vi "Bracket Deletion.vi"(0 "string input with brackets":string, 1 "error in (no error)":errorcluster) -> (2 "string output balanced":string, 3 "string output rest":string, 4 "error out":errorcluster)   [LabVIEW 2020, in "NI_Gmath.lvlib"]
uses:
  <vilib>/gmath/NI_Gmath.lvlib
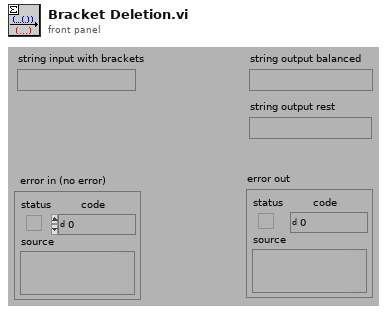
[diagram p1: front panel]
types:
  T1 = cluster{bool, i32, "string input with brackets":string}
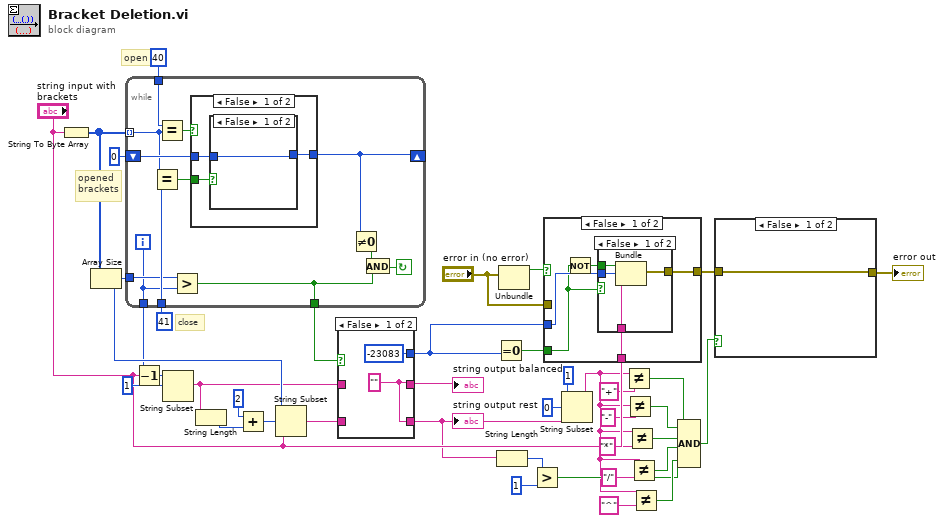
[diagram p0: block diagram]
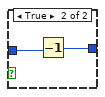
[diagram p2: hidden frame]
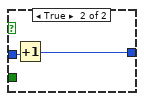
[diagram p3: hidden frame]
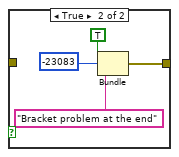
[diagram p4: hidden frame]
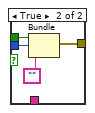
[diagram p5: hidden frame]
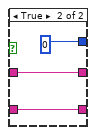
[diagram p7: hidden frame]
diagram:
  # "close"
  # "open"
  # "opened\nbrackets"
  n1 = String To Byte Array(string="string input with brackets") -> (unsigned byte array=w37:u8[])
  n2 = Array Size(array=w37) -> (size(s)=w36:i32)
  n3 = while {
    tunnel: [w41] -> w33
    tunnel: [w42] -> w25
    tunnel: w36 -> [w45]
    tunnel: 41 -> [w49]
    tunnel: 40 -> [w52]
    tunnel: w37 -> [w48] mode=indexing
    shift-left: 0 -> [w50]
    shift-right: [w46] -> _
    i -> [w41]
    stop <- w43 continue-if-true
    n4 = Equal?(x=w48, y=w49) -> (x = y?=w47:bool)
    n5 = Equal?(x=w52, y=w48) -> (x = y?=w51:bool)
    n6 = Greater?(x=w45, y=w41) -> (0:w42:bool)
    n7 = case shown="False" w51 {
      tunnel: w50 -> [w54 w60]
      tunnel: [w53 w59] -> w46
      tunnel: w47 -> [w55 _]
      frame False {
        n8 = case shown="False" w55 {
          tunnel: w54 -> [w56 w58]
          tunnel: [w56 w57] -> w53
          frame False {
          }
          frame True {
            n9 = Decrement(x=w58) -> (x-1=w57:i32)
          }
        }
      }
      frame True {
        n10 = Increment(x=w60) -> (x+1=w59:i32)
      }
    }
    n11 = Not Equal To 0?(x=w46) -> (x != 0?=w44:bool)
    n12 = And(x=w44, y=w42) -> (x .and. y?=w43:bool)
  }
  n13 = Decrement(x=w33) -> (x-1=w31:i32)
  n14 = String Subset(string="string input with brackets", offset (0)=1, length (rest)=w31) -> (substring=w35:string)
  n15 = String Length(string=w35) -> (length=w30:i32)
  n16 = Add(x=2, y=w30) -> (x+y=w28:i32)
  n17 = String Subset(string="string input with brackets", offset (0)=w28, length (rest)=w36) -> (substring=w34:string)
  n18 = case shown="False" w25 {
    tunnel: [-23083 0] -> w24
    tunnel: w35 -> [_ w64]
    tunnel: [w61 w64] -> w23
    tunnel: w34 -> [_ w63]
    tunnel: [w61 w63] -> w20
    frame False {
      w61 = ""
    }
    frame True {
    }
  }
  "string output balanced" <- w23
  "string output rest" <- w20
  n19 = Equal To 0?(x=w24) -> (x = 0?=w22:bool)
  n20 = String Length(string=w20) -> (length=w19:i32)
  n21 = Unbundle("error in (no error)") -> ("status"=w27:bool)  [unwired: 2 out]
  n22 = Greater?(x=w19, y=1) -> (0:w5:bool)
  n23 = case shown="False" w27 {
    tunnel: "error in (no error)" -> [_ w79]
    tunnel: [w70 w79] -> w2
    tunnel: w24 -> [w69 _]
    tunnel: w22 -> [w68 _]
    tunnel: "string input with brackets" -> [w67 _]
    frame False {
      n24 = Not(x=w68) -> (.not. x?=w66:bool)
      n25 = case shown="False" w68 {
        tunnel: w69 -> [w74 w78]
        tunnel: w66 -> [w73 w77]
        tunnel: [w72 w76] -> w70
        tunnel: w67 -> [w71 _]
        frame False {
          n26 = Bundle(w73, w74, "string input with brackets"=w71) -> (w72:T1)  [unwired: 1 in]
        }
        frame True {
          n27 = Bundle(w77, w78, "") -> (w76:errorcluster)  [unwired: 1 in]
        }
      }
    }
    frame True {
    }
  }
  n28 = String Subset(string=w20, offset (0)=0, length (rest)=1 ("length")) -> (substring=w1:string)
  n29 = Not Equal?(x=w1, y="+") -> (x != y?=w10:bool)
  n30 = Not Equal?(x=w1, y="-") -> (x != y?=w9:bool)
  n31 = Not Equal?(x=w1, y="*") -> (x != y?=w8:bool)
  n32 = Not Equal?(x=w1, y="/") -> (x != y?=w7:bool)
  n33 = Not Equal?(x=w1, y="^") -> (x != y?=w6:bool)
  n34 = Compound Arithmetic op=AND(w10, w9, w8, w7, w6, w5) -> (w4:bool)
  n35 = case shown="False" w4 {
    tunnel: [w80 w82] -> w3
    tunnel: w2 -> [w80 _]
    frame False {
    }
    frame True {
      n36 = Bundle(TRUE, -23083, "Bracket problem at the end") -> (w82:errorcluster)  [unwired: 1 in]
    }
  }
  "error out" <- w3
